vi "Zadanie7_3_done.vi"() -> ()   [LabVIEW 2012]
panel:
  in  "Naciśnij aby rozpocząć działanie programu":bool
  out "Użytkownik:":string
  in  "Wartość kąta a":dbl(knob) scale=0.0..90.0
  in  "Amplituda x = A":dbl
  in  "Wartość kąta b":dbl(knob) scale=0.0..90.0
  in  "Amplituda y = B":dbl
  in  "stop":bool
  in  "resetuj wejście x":bool
  in  "resetuj wejście y":bool
  out "wykres krzywych Lissajous":cluster{"Y":dbl[], "Y":dbl[]}[](graph)
  # "Program pozwala obserwować symulacje krzywych Lissajous \ndla podanych wartości kąta i amplitudy. \nDodatkowo umożliwa resetowanie wartości wejściowych"
  # "x(t) = A sin(a(t))"
  # "y(t) = B sin(b(t))"
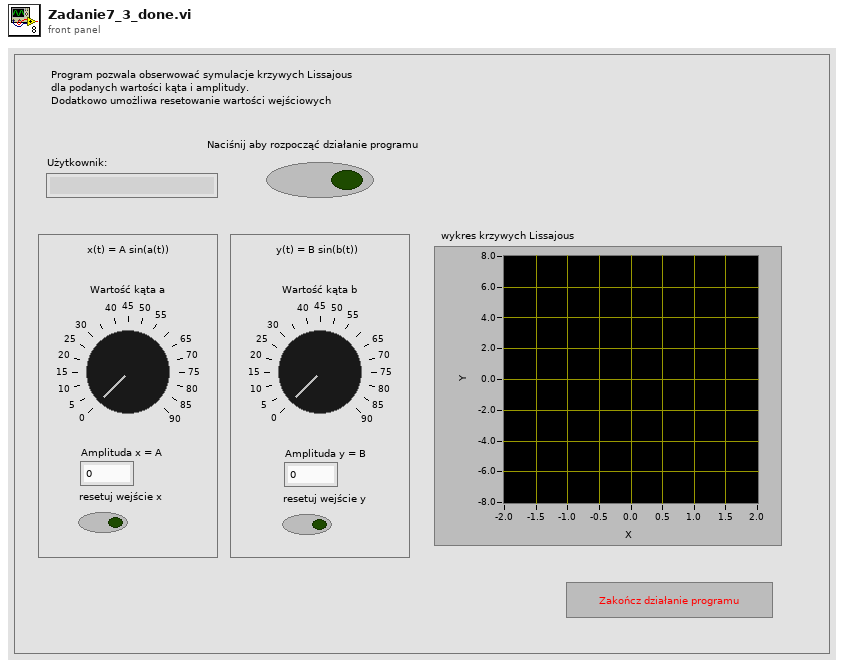
[diagram p1: front panel]
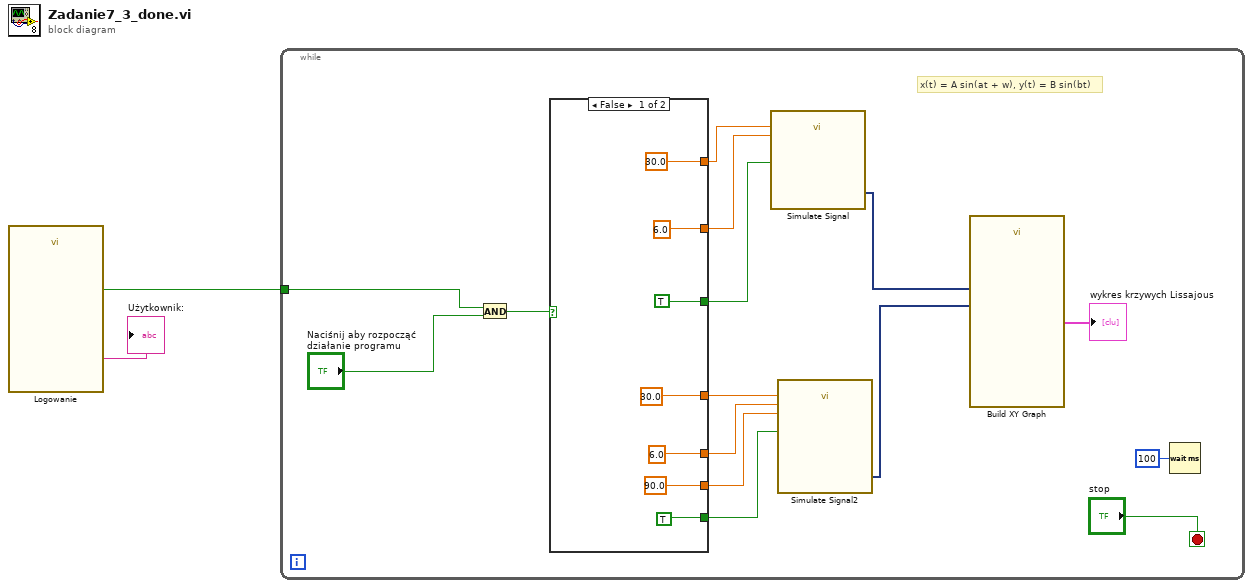
[diagram p0: block diagram]
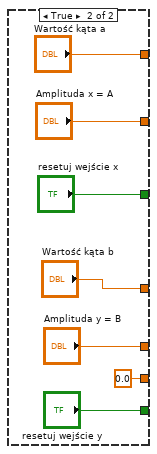
[diagram p2: hidden frame]
diagram:
  n1 = call "Logowanie"() -> ("Podaj nazwę:"=→"Użytkownik:":string, "Dalej"=w1:bool)  [unwired: 16 in, 2 out]
  n2 = while {
    tunnel: w1 -> [w4]
    stop <- "stop" stop-if-true
    # "x(t) = A sin(at + w), y(t) = B sin(bt)"
    n3 = And(x=w4, y="Naciśnij aby rozpocząć działanie programu") -> (x .and. y?=w3:bool)
    n4 = case shown="False" w3 {
      tunnel: [TRUE ("reet_signal1") "resetuj wejście x"] -> w12
      tunnel: [6.0 ("Offset") "Amplituda x = A"] -> w11
      tunnel: [30.0 ("Frequency") "Wartość kąta a"] -> w10
      tunnel: [30.0 ("Offset") "Wartość kąta b"] -> w9
      tunnel: [6.0 ("Frequency") "Amplituda y = B"] -> w8
      tunnel: [TRUE ("reet_signal1") "resetuj wejście y"] -> w7
      tunnel: [90.0 ("Offset") 0.0 ("Offset")] -> w6
      frame False {
      }
      frame True {
      }
    }
    n5 = call "Simulate Signal"("Reset Signal"=w12, "Frequency"=w10, "Amplitude"=w11) -> ("Sine one"=w15:dynamicdata)  [unwired: 11 in, 1 out]
    n6 = call "Simulate Signal2"("Reset Signal"=w7, "Frequency"=w9, "Amplitude"=w8, "Phase"=w6) -> ("Sine two"=w14:dynamicdata)  [unwired: 10 in, 1 out]
    n7 = call "Build XY Graph"("Y Input"=w14, "X Input"=w15) -> ("XY Graph"=→"wykres krzywych Lissajous":cluster{"Y":dbl[], "Y":dbl[]}[])  [unwired: 3 in, 6 out]
    n8 = Wait (ms)(milliseconds to wait=u32 100) -> ()  [unwired: 1 out]
  }
